vi "speed.vi"(1 "Knob":i32(knob) scale=0.0..2.0) -> (0 "Speed":dbl(knob) scale=0.0..5.0)   [LabVIEW 2013]
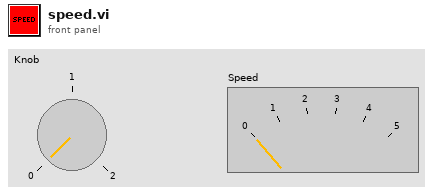
[diagram p1: front panel]
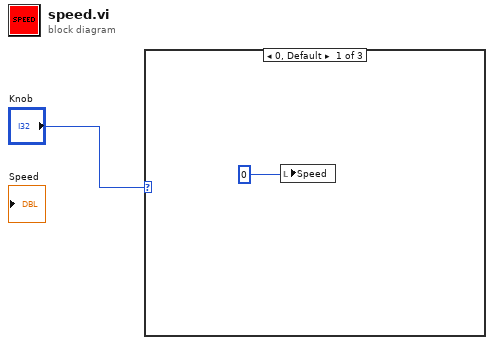
[diagram p0: block diagram]
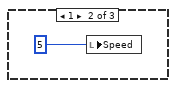
[diagram p2: hidden frame]
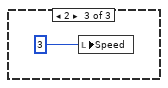
[diagram p3: hidden frame]
diagram:
  n1 = case shown="0, Default" "Knob" {
    frame 0, Default {
      n2 = local write "Speed"(0) -> ()
    }
    frame 1 {
      n3 = local write "Speed"(5) -> ()
    }
    frame 2 {
      n4 = local write "Speed"(3) -> ()
    }
  }
